vi "Weather Station UI.vi"(7 "stop":bool, 9 "Lower Limit":dbl=10.0 min=0.0 max=50.0, 10 "Upper Limit":dbl=30.0 min=0.0 max=50.0) -> (1 "Warning":string, 2 "Temperature History":dbl(graph))   [LabVIEW 2010]
doc: "This is the main VI in the Weather Station Project. It contains the user interface for a temperature warning system. Temperature is retrieved every half second; data is logged when a warning has occurred.\n\nUser inputs: Temperature Upper Limit, Temperature Lower Limit, Temperature Units.\nOutputs: Current Temperature, Warning State"
uses:
  Supporting Files/Weather Station States.ctl
  Instance           1 26Saved   Weather Station UI .vi
panel:
  # "Temperature Ranges (C)"
  # "Heat \nStroke"
  # "Freeze"
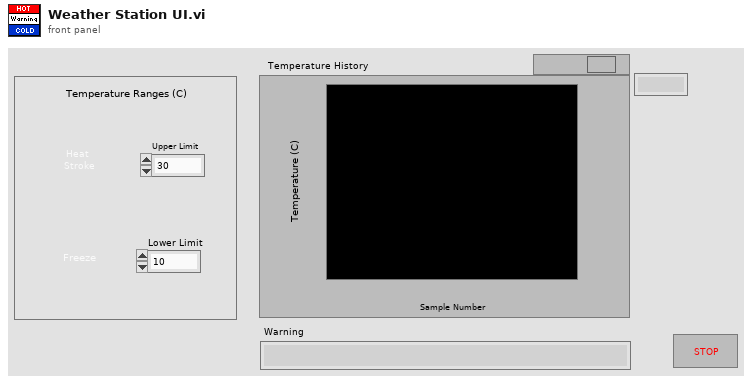
[diagram p1: front panel]
types:
  T1 = enum16{"open", "replace", "create", "open or create", "replace or create", "replace or create with confirmation"}
  T2 = typedef "Weather Station States.ctl" = enum16{"Acquisition", "Analysis", "Data Log", "Time Check"}
  T3 = cluster{"Temperature":dbl, "T Upper Limit":dbl, "T Lower Limit":dbl, "Warning":string}
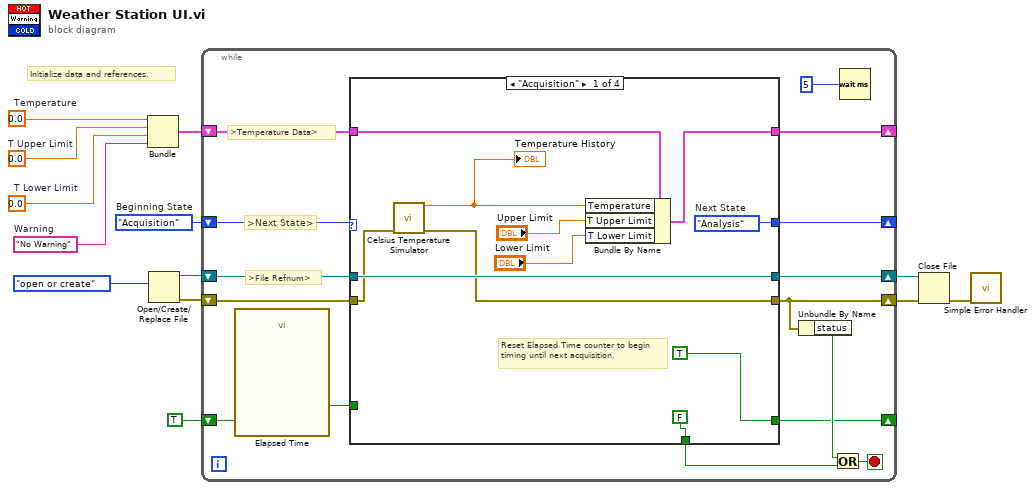
[diagram p0: block diagram]
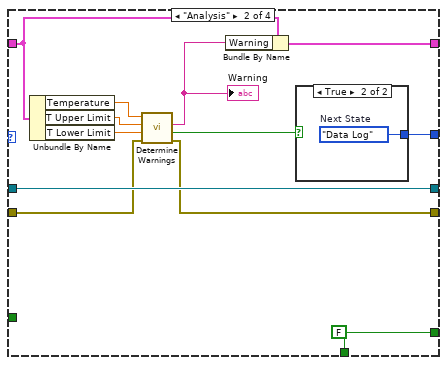
[diagram p2: hidden frame]
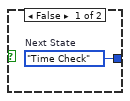
[diagram p3: hidden frame]
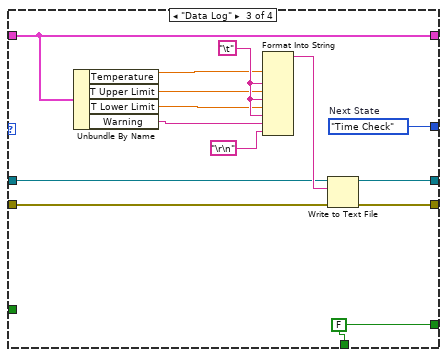
[diagram p4: hidden frame]
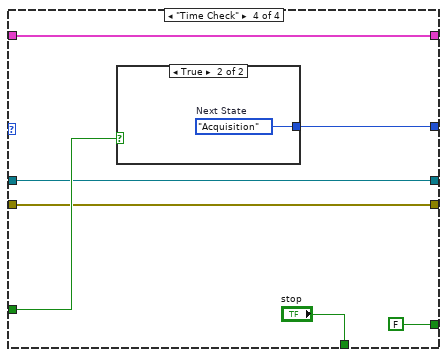
[diagram p5: hidden frame]
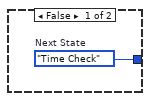
[diagram p6: hidden frame]
diagram:
  w7 = 0.0  # T Lower Limit
  w6 = 0.0  # T Upper Limit
  w8 = "No Warning"  # Warning
  w4 = 0.0  # Temperature
  w13 = Weather_Station_States."Acquisition"  # Beginning State
  # "Initialize data and references."
  n1 = Bundle("Temperature"=w4, "T Upper Limit"=w6, "T Lower Limit"=w7, "Warning"=w8) -> (w1:T3)  [unwired: 1 in]
  n2 = Open/Create/Replace File(operation (0:open)=T1."open or create") -> (refnum out=w3:refnum<file>, error out=w2:errorcluster)  [unwired: 5 in, 1 out]
  n3 = while {
    shift-right: [w27] -> _
    shift-left: w13 -> [w28]
    shift-right: [w24] -> w12
    shift-left: w2 -> [w26]
    shift-right: [w14] -> _
    shift-left: w1 -> [w21]
    shift-right: [w22] -> w11
    shift-left: w3 -> [w20]
    shift-right: [w15] -> _
    shift-left: TRUE ("stop") -> [w17]
    stop <- w25 stop-if-true
    # ">Temperature Data>"
    # ">File Refnum>"
    # ">Next State>"
    n4 = call "Elapsed Time"("Reset"=w17) -> ("Time has Elapsed"=w16:bool)  [unwired: 11 in, 7 out]
    n5 = case shown="\"Acquisition\"" w28 {
      tunnel: [w39 w49 w67 w73] -> w27
      tunnel: [w29 w42 w65 w69] -> w24
      tunnel: w26 -> [w30 w43 w66 w69]
      tunnel: [w38 w51 w64 w70] -> w22
      tunnel: [w32 w44 w54 w68] -> w14
      tunnel: w21 -> [w35 w45 w54 w68]
      tunnel: w20 -> [w38 w51 w62 w70]
      tunnel: [FALSE ("stop") w50 w60 "stop"] -> w19
      tunnel: w16 -> [_ _ _ w74]
      tunnel: [TRUE ("stop") w50 w60 FALSE ("stop")] -> w15
      frame "Acquisition" {
        w39 = Weather_Station_States."Analysis"  # Next State
        # "Reset Elapsed Time counter to begin timing until next acquisition."
        n6 = call "Celsius Temperature Simulator.vi"("error in (no error)"=w30) -> ("Temperature"=w31:dbl, "error out"=w29:errorcluster)  [unwired: 13 in]
        "Temperature History" <- w31
        n7 = Bundle By Name(cluster=w35, "Temperature"=w31, "T Upper Limit"="Upper Limit", "T Lower Limit"="Lower Limit") -> (w32:T3)
      }
      frame "Analysis" {
        w50 = FALSE ("stop")
        n8 = Unbundle By Name(w45) -> ("Temperature"=w48:dbl, "T Upper Limit"=w47:dbl, "T Lower Limit"=w46:dbl)
        n9 = call "Determine Warnings.vi"("error in (no error)"=w43, "Min Temp"=w46, "Max Temp"=w47, "Current Temp"=w48) -> ("error out"=w42:errorcluster, "Warning?"=w40:bool, "Warning Text"=w41:string)  [unwired: 5 in]
        "Warning" <- w41
        n10 = Bundle By Name(cluster=w45, "Warning"=w41) -> (w44:T3)
        n11 = case shown="True" w40 {
          tunnel: [w52 w53] -> w49
          frame False {
            w52 = Weather_Station_States."Time Check"  # Next State
          }
          frame True {
            w53 = Weather_Station_States."Data Log"  # Next State
          }
        }
      }
      frame "Data Log" {
        w67 = Weather_Station_States."Time Check"  # Next State
        w60 = FALSE ("stop")
        w61 = "\t"
        n12 = Unbundle By Name(w54) -> ("Temperature"=w59:dbl, "T Upper Limit"=w58:dbl, "T Lower Limit"=w57:dbl, "Warning"=w56:string)
        n13 = Format Into String(w59, w61, w58, w61, w57, w61, w56, "\r\n") -> (resulting string=w63:string)  [unwired: 3 in, 1 out]
        n14 = Write to Text File(file (use dialog)=w62, text=w63, error in=w66) -> (refnum out=w64:refnum<file>, error out=w65:errorcluster)  [unwired: 1 in, 1 out]
      }
      frame "Time Check" {
        n15 = case shown="True" w74 {
          tunnel: [w75 w76] -> w73
          frame False {
            w75 = Weather_Station_States."Time Check"  # Next State
          }
          frame True {
            w76 = Weather_Station_States."Acquisition"  # Next State
          }
        }
      }
    }
    n16 = Unbundle By Name(w24) -> ("status"=w23:bool)
    n17 = Or(x=w23, y=w19) -> (x .or. y?=w25:bool)
    n18 = Wait (ms)(milliseconds to wait=u32 5 ("y")) -> ()  [unwired: 1 out]
  }
  n19 = Close File(refnum=w11, error in=w12) -> (error out=w10:errorcluster)  [unwired: 1 out]
  n20 = call <vilib>:"Simple Error Handler.vi"("error in (no error)"=w10) -> ()  [unwired: 4 in, 5 out]
